vi "Server.vi"() -> ()   [LabVIEW 2009]
uses:
  <userlib>/_OpenG.lib/appcontrol/appcontrol.llb/Close Generic Object Refnum (Array VI)__ogtk.vi
  <vilib>/Utility/config.llb/NI_LVConfig.lvlib
panel:
  out "Exec.State":T1(ring)=enum."Run top level"
  in  "stop":bool
  in  "Controllers":i32(listbox)=5
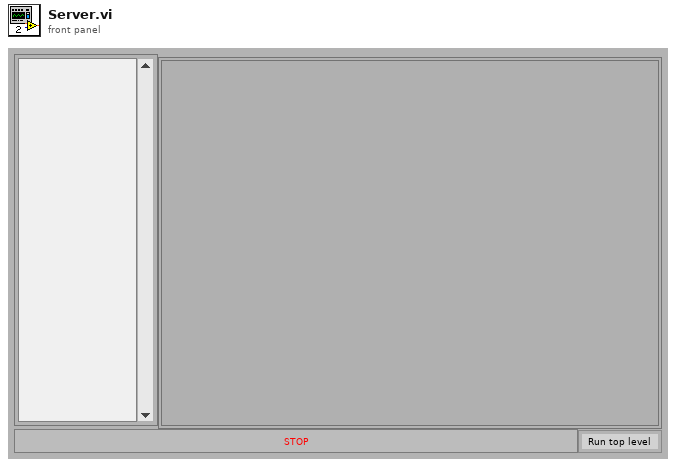
[diagram p1: front panel]
types:
  T1 = enum32{"Bad", "Idle", "Run top level", "Running"}
  T2 = typedef "NI_LVConfig.lvlib/Config Data RefNum.ctl" = refnum<k1>
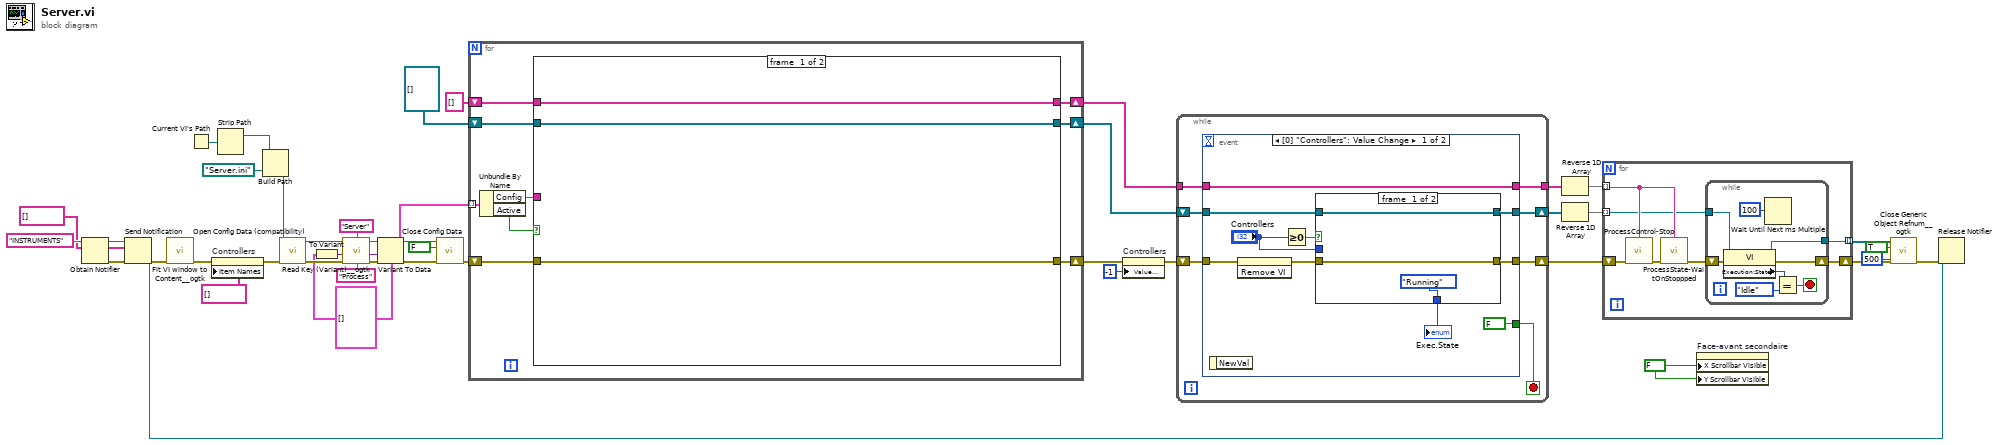
[diagram p0: block diagram]
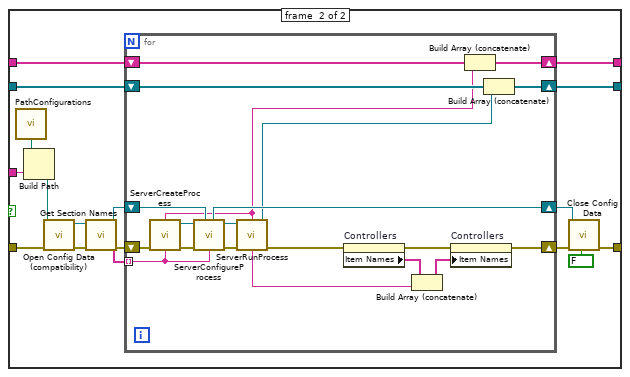
[diagram p2: hidden frame]
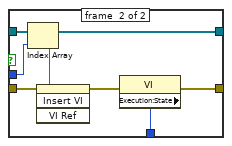
[diagram p3: hidden frame]
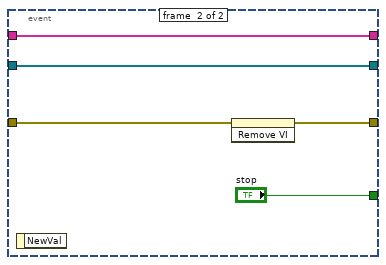
[diagram p4: hidden frame]
diagram:
  w1 = string[] []
  w19 = cluster{"Config":string, "Active":bool}[] []
  w37 = FALSE ("Barre de défil. X visible")
  n1 = Obtain Notifier(name (unnamed)="INSTRUMENTS", notification data type=w1) -> (notifier out=w3:refnum<notifier>, error out=w5:errorcluster)  [unwired: 2 in, 1 out]
  n2 = Send Notification(notification=w1, notifier=w3, error in (no error)=w5) -> (notifier out=w2:refnum<notifier>, error out=w4:errorcluster)
  n3 = call <userlib>:"Fit VI window to Content__ogtk.vi"("error in (no error)"=w4) -> ("error out"=w26:errorcluster)  [unwired: 2 in, 4 out]
  n4 = Current VI's Path() -> (path=w32:path)
  n5 = property on="Controllers" class="ListeDéroulante (strict)"(error in=w26, "Item Names"=string[] [] ("Noms éléments")) -> (error out=w27:errorcluster)  [unwired: 1 in, 1 out]
  n6 = Strip Path(path=w32) -> (stripped path=w29:path)  [unwired: 1 out]
  n7 = Build Path(base path=w29, name or relative path=path "Server.ini" ("configuration file path")) -> (appended path=w24:path)
  n8 = call <vilib>:"Open Config Data (compatibility).vi"("error in (no error)"=w27, "configuration file path"=w24) -> ("error out"=w33:errorcluster, "refnum"=w34:T2)  [unwired: 7 in, 1 out]
  n9 = To Variant(anything=w19) -> (Variant=w22:variant)
  n10 = call <userlib>:"Read Key (Variant)__ogtk.vi"("section"="Server", "error in (no error)"=w33, "type"=w22, "key (optional)"="Process" ("key"), "refnum"=w34) -> ("error out"=w20:errorcluster, "key-value"=w21:variant, "refnum out"=w18:T2)  [unwired: 4 out]
  n11 = Variant To Data(error in=w20, Variant=w21, type=w19) -> (error out=w17:errorcluster, data=w15:cluster{"Config":string, "Active":bool}[])
  n12 = call <vilib>:"Close Config Data.vi"("error in (no error)"=w17, "write file if changed (T)"=FALSE ("write configuration file? (T)"), "refnum"=w18) -> ("error out"=w16:errorcluster)  [unwired: 8 out]
  n13 = for {
    shift-right: [w53] -> w44
    shift-left: w16 -> [w52]
    tunnel: w15 -> [w51] mode=indexing
    shift-right: [w45] -> w12
    shift-left: refnum<vi>[] [] -> [w48]
    shift-right: [w46] -> w13
    shift-left: string[] [] -> [w47]
    n14 = Unbundle By Name(w51) -> ("Config"=w49:string, "Active"=w50:bool)
    n15 = case shown="True" w50 {
      tunnel: [w54 w69] -> w53
      tunnel: w52 -> [w54 w67]
      tunnel: w49 -> [_ w66]
      tunnel: w48 -> [w55 w65]
      tunnel: w47 -> [w56 w64]
      tunnel: [w56 w63] -> w46
      tunnel: [w55 w62] -> w45
      frame #0 {
      }
      frame #1 {
        n16 = call "PathConfigurations.vi"() -> ("OhanaOS Path"=w57:path)
        n17 = Build Path(base path=w57, name or relative path=w66) -> (appended path=w68:path)
        n18 = call <vilib>:"Open Config Data (compatibility).vi"("error in (no error)"=w67, "configuration file path"=w68) -> ("error out"=w72:errorcluster, "refnum"=w73:T2)  [unwired: 7 in, 1 out]
        n19 = call <vilib>:"Get Section Names.vi"("error in (no error)"=w72, "refnum"=w73) -> ("error out"=w71:errorcluster, "section names"=w60:string[], "refnum out"=w59:T2)  [unwired: 7 out]
        n20 = for {
          shift-right: [w88] -> w70
          shift-left: w71 -> [w90]
          shift-right: [w77] -> w58
          shift-left: w59 -> [w78]
          shift-right: [w83] -> w62
          shift-left: w65 -> [w82]
          shift-right: [w84] -> w63
          shift-left: w64 -> [w85]
          tunnel: w60 -> [w79] mode=indexing
          n21 = call "ServerCreateProcess.vi"("Process Header"=w79, "error in (no error)"=w90) -> ("Process Reference"=w81:refnum<vi>, "Process Name"=w74:string, "error out"=w91:errorcluster)  [unwired: 3 in, 2 out]
          n22 = call "ServerConfigureProcess.vi"("error out"=w91, "Process Header"=w79, "Process Reference in"=w81, "ConfigFile Reference in"=w78) -> ("entrée d'erreur (pas d'erreur)"=w80:errorcluster, "ConfigFile Reference out"=w77:T2, "Process Reference out"=w76:refnum<vi>)  [unwired: 4 out]
          n23 = call "ServerRunProcess.vi"("Process Name"=w74, "Process Reference in"=w76, "Error in (no error)"=w80) -> ("Process Reference out"=w75:refnum<vi>, "Error out"=w89:errorcluster)  [unwired: 1 in, 4 out]
          n24 = property on="Controllers" class="ListeDéroulante (strict)"(error in=w89) -> (error out=w88:errorcluster, "Item Names"=w87:string[])  [unwired: 1 in, 1 out]
          n25 = Build Array (concatenate)(w87, w74) -> (w86:string[])
          n26 = property on="Controllers" class="ListeDéroulante (strict)"("Item Names"=w86) -> ()  [unwired: 2 in, 2 out]
          n27 = Build Array (concatenate)(w85, w74) -> (w84:string[])
          n28 = Build Array (concatenate)(w82, w75) -> (w83:refnum<vi>[])
        }
        n29 = call <vilib>:"Close Config Data.vi"("error in (no error)"=w70, "write file if changed (T)"=FALSE ("write configuration file? (T)"), "refnum"=w58) -> ("error out"=w69:errorcluster)  [unwired: 8 out]
      }
    }
  }
  n30 = property on="Controllers" class="ListeDéroulante (strict)"(error in=w44, "Value (Signaling)"=-1 ("Valeur (Signalisation)")) -> (error out=w42:errorcluster)  [unwired: 1 in, 1 out]
  n31 = while {
    shift-right: [w95] -> w40
    shift-left: w42 -> [w98]
    shift-right: [w94] -> w9
    shift-left: w12 -> [w97]
    tunnel: [w92] -> w10
    tunnel: w13 -> [w93]
    stop <- w96 stop-if-true
    n32 = event shown="[0] \"Controllers\": Value Change" {
      selector: _ -> [_ _]
      dyn-events: _ -> [_ _]
      timeout: _ -> [_ _]
      tunnel: w98 -> [w108 w122]
      tunnel: w97 -> [w103 w120]
      tunnel: [FALSE ("stop") "stop"] -> w96
      tunnel: [w106 w121] -> w95
      tunnel: [w101 w120] -> w94
      tunnel: [w99 w119] -> w92
      tunnel: w93 -> [w99 w119]
      event #0 {
        n33 = event-data() -> ()  [unwired: 2 out]
        n34 = invoke on="Face-avant secondaire" class="Face-avantSecondaire" method="Remove VI"(error in=w108) -> (error out=w107:errorcluster)  [unwired: 2 in, 2 out]
        n35 = Greater Or Equal To 0?(x="Controllers") -> (x >= 0?=w102:bool)
        n36 = case shown="True" w102 {
          tunnel: w107 -> [w111 w118]
          tunnel: [w111 w114] -> w106
          tunnel: "Controllers" -> [_ w117]
          tunnel: w103 -> [w110 w116]
          tunnel: [w110 w116] -> w101
          tunnel: [T1."Running" ("Exec.State") w113] -> w100
          frame #0 {
          }
          frame #1 {
            n37 = Index Array(array=w116, index=w117) -> (element=w112:refnum<vi>)
            n38 = invoke on="Face-avant secondaire" class="Face-avantSecondaire" method="Insert VI"(error in=w118, "VI Ref"=w112) -> (error out=w115:errorcluster)  [unwired: 2 in, 3 out]
            n39 = property class="VI"(error in=w115) -> (error out=w114:errorcluster, "Execution:State"=w113:T1)  [unwired: 1 in, 1 out]
          }
        }
        "Exec.State" <- w100
      }
      event #1 {
        n40 = event-data() -> ()  [unwired: 2 out]
        n41 = invoke on="Face-avant secondaire" class="Face-avantSecondaire" method="Remove VI"(error in=w122) -> (error out=w121:errorcluster)  [unwired: 2 in, 2 out]
      }
    }
  }
  n42 = Reverse 1D Array(array=w10) -> (reversed array=w28:string[])
  n43 = Reverse 1D Array(array=w9) -> (reversed array=w36:refnum<vi>[])
  n44 = for {
    tunnel: w36 -> [w126] mode=indexing
    shift-right: [w130] -> w38
    shift-left: w40 -> [w128]
    tunnel: [w129] -> w39 mode=indexing
    tunnel: w28 -> [w127] mode=indexing
    n45 = call "ProcessControl-Stop.vi"("PROCESS"=w127, "error in (no error)"=w128) -> ("error out"=w125:errorcluster)  [unwired: 7 out]
    n46 = call "ProcessState-WaitOnStoppped.vi"("PROCESS"=w127, "error in (no error)"=w125) -> ("error out"=w124:errorcluster)  [unwired: 7 out]
    n47 = while {
      shift-right: [w133] -> w130
      shift-left: w124 -> [w134]
      tunnel: [w132] -> w129
      tunnel: w126 -> [w131]
      stop <- w136 stop-if-true
      n48 = property class="VI"(reference=w131, error in=w134) -> (reference out=w132:refnum<vi>, error out=w133:errorcluster, "Execution:State"=w138:T1)
      n49 = Wait Until Next ms Multiple(millisecond multiple=u32 100 ("n millisecondes")) -> ()  [unwired: 1 out]
      n50 = Equal?(x=w138, y=T1."Idle") -> (x = y?=w136:bool)
    }
  }
  n51 = property on="Face-avant secondaire" class="Face-avantSecondaire"("X Scrollbar Visible"=w37, "Y Scrollbar Visible"=w37) -> ()  [unwired: 2 in, 2 out]
  n52 = call-poly <userlib>:"Close Generic Object Refnum__ogtk.vi"("error in (no error)"=w38, "timeout in ms (-1)"=500 ("timeout (ms)"), "wait on unloaded? (FALSE)"=TRUE, "Gen Refnum Array"=w39) -> ("error out"=w6:errorcluster)  [unwired: 7 out]
  n53 = Release Notifier(notifier=w2, error in (no error)=w6) -> ()  [unwired: 4 out]
